vi "Create FP Item.vi"(6 "Cluster Component":bool, 8 "error in (no error)":errorcluster, 10 "GObject In":refnum<vi>, 11 "Graph in":refnum<class "Graph.lvclass">) -> (0 "error out":errorcluster, 1 "Is Control":bool, 2 "Is Indicator":bool, 3 "Graph out":refnum<class "Graph.lvclass">, 4 "All Objects Created":refnum<class "Object.lvclass">[](array[class]), 5 "Is Visible":bool)   [LabVIEW 2017, in "Front Panel Publisher.lvlib" / "Graph.lvclass"]
uses:
  Graph.lvclass
  Attributes.ctl
  Control_class/Control.lvclass
  Object_class/Object.lvclass
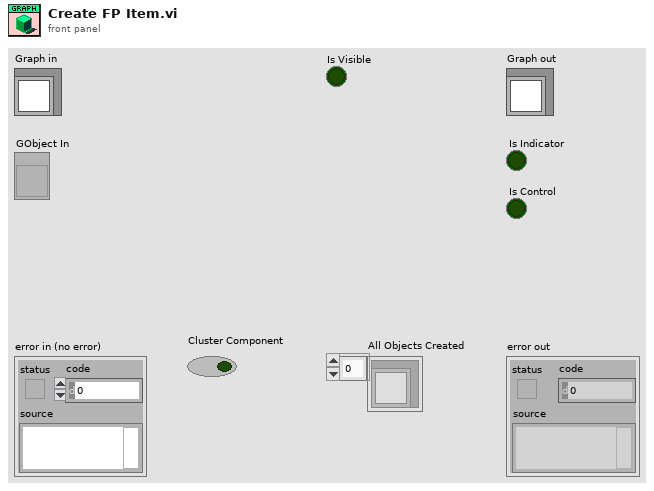
[diagram p1: front panel]
types:
  T1 = typedef "Front Panel Publisher.lvlib/Graph.lvclass/Attributes.ctl" = cluster{"X Label Text":string, "X Format String":string, "Y Label Text":string[], "Y Format String":string[], "Plot Y Axis Selection":enum16{"Y Axis", "Y2 Axis"}[], "Width":u32, "Series JSON Data":string}
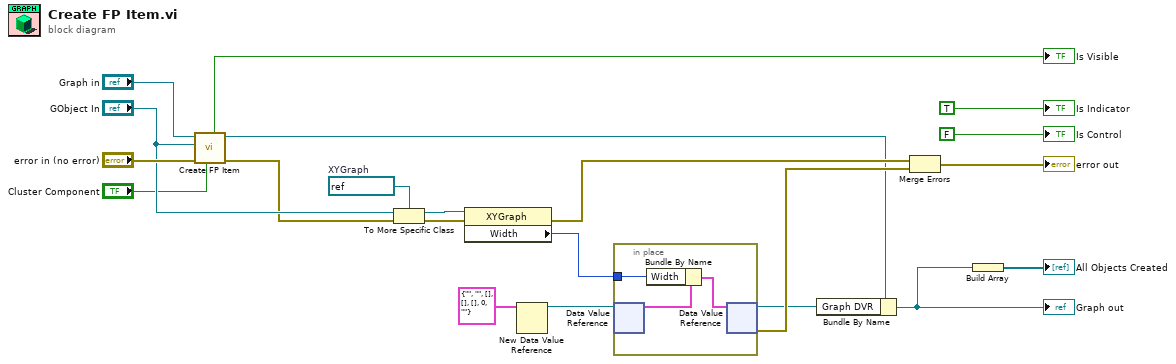
[diagram p0: block diagram]
diagram:
  w18 = refnum<vi> refnum  # XYGraph
  n1 = call-parent "Create FP Item.vi"("Cluster Component"="Cluster Component", "error in (no error)"="error in (no error)", "GObject In"="GObject In", "GControl in"="Graph in") -> ("error out"=w14:errorcluster, "GControl out"=w5:refnum<class "Graph.lvclass">, "Is Visible"=→"Is Visible":bool)  [unwired: 2 in, 3 out]
  n2 = To More Specific Class(target class=w18, reference="GObject In", error in=w14) -> (specific class reference=w17:refnum<vi>, error out=w16:errorcluster)
  n3 = property class="XYGraph"(reference=w17, error in=w16) -> (error out=w13:errorcluster, "Width"=w10:u32)  [unwired: 1 out]
  n4 = New Data Value Reference(data value=T1 {"X Label Text"="", "X Format String"="", "Y Label Text"=[], "Y Format String"=[], "Plot Y Axis Selection"=[], "Width"=0, "Series JSON Data"=""}) -> (data value reference=w6:refnum<data-value>)  [unwired: 1 in, 1 out]
  n5 = in-place {
    in-place-border: w10 -> [w22]
    n6 = in-place-dvr #1(w6) -> (w24:T1)  [unwired: 1 out]
    n7 = Bundle By Name(cluster=w24, "Width"=w22) -> (w23:T1)
    n8 = in-place-dvr #1(w23) -> (w4:refnum<data-value>, w8:errorcluster)
  }
  n9 = Bundle By Name(cluster=w5, "Graph DVR"=w4) -> (w2:refnum<class "Graph.lvclass">)
  "Graph out" <- w2
  n10 = Merge Errors(w13, w8) -> (→"error out":errorcluster)
  n11 = Build Array(w2) -> (→"All Objects Created":refnum<class "Graph.lvclass">[])
  "Is Indicator" <- TRUE ("Is Indicator")
  "Is Control" <- FALSE ("Is Control")
